vi "Untitled 2.vi"() -> ()   [LabVIEW 2017]
uses:
  <vilib>/addons/internet/NI_InternetTK_Core_VIs.lvlib
panel:
  out "concatenated string 2":string
  out "concatenated string":string
  out "content":string
  in  "Machine":string="STC1250"
  in  "MT Connect Agent":string="http://amrcmtconnect.shef.ac.uk:5000/"
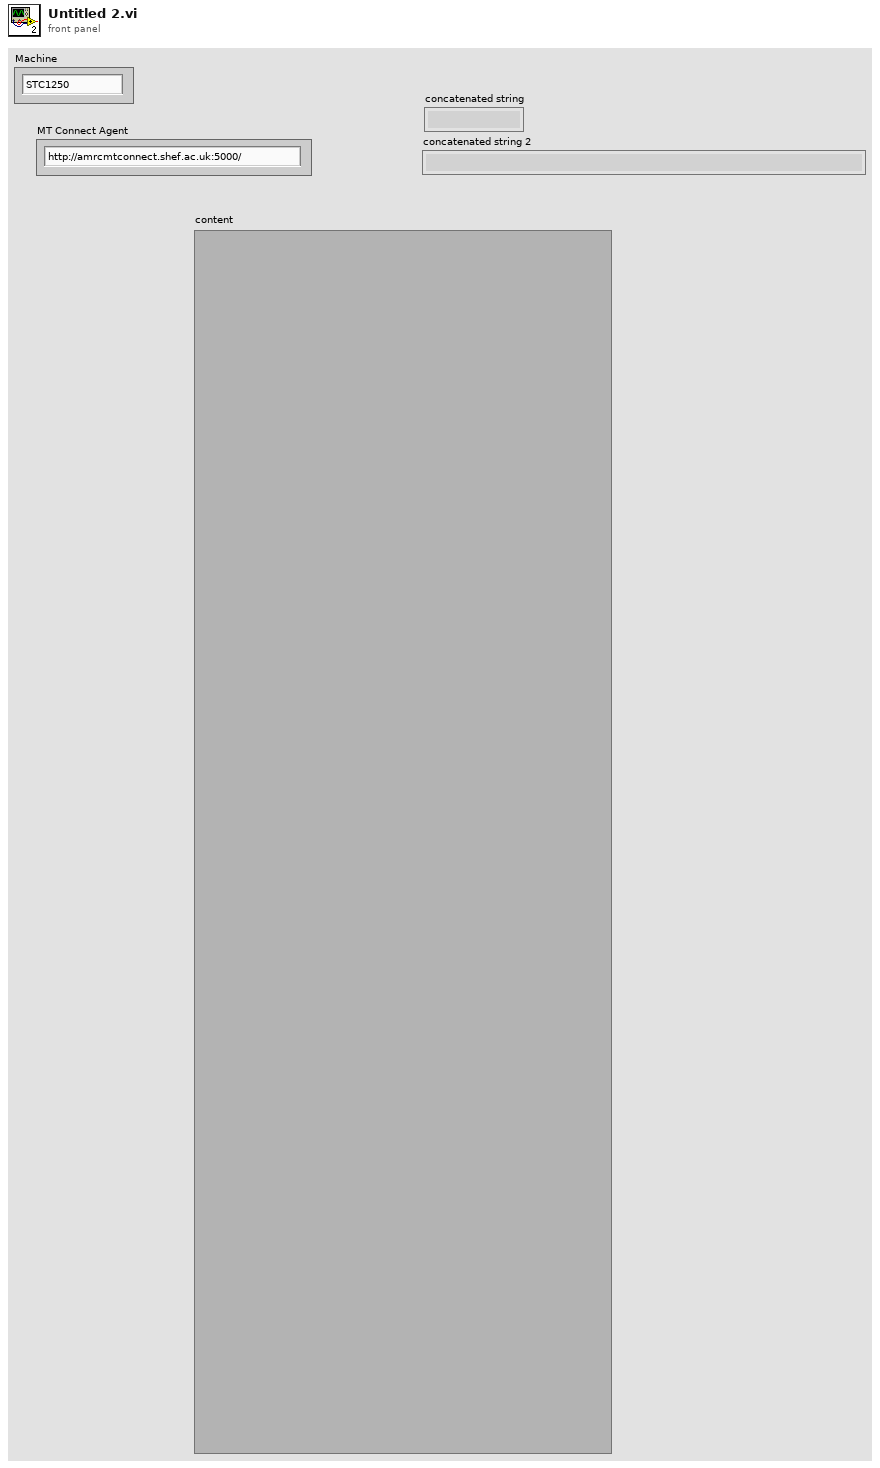
[diagram p1: front panel]
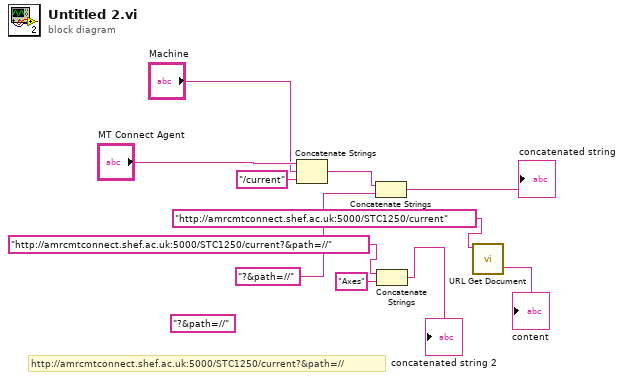
[diagram p0: block diagram]
diagram:
  (unwired) "?&path=//" ("string")
  # "http://amrcmtconnect.shef.ac.uk:5000/STC1250/current?&path=//"
  n1 = Concatenate Strings("MT Connect Agent", "Machine", "/current" ("string")) -> (w8:string)
  n2 = Concatenate Strings(w8, "?&path=//" ("string")) -> (→"concatenated string":string)
  n3 = Concatenate Strings("http://amrcmtconnect.shef.ac.uk:5000/STC1250/current?&path=//" ("URL"), "Axes" ("string")) -> (→"concatenated string 2":string)
  n4 = call <vilib>:"URL Get Document.vi"("URL"="http://amrcmtconnect.shef.ac.uk:5000/STC1250/current") -> ("content"=→"content":string)  [unwired: 6 in, 4 out]
